vi "Save_Ensight.vi"() -> (5 "Plug in titles":string[](array[string]), 7 "Plug in values":string[](array[string]))   [LabVIEW 2011]
uses:
  Globals/LDA_meas_global_1.vi
  Globals/Plug_in_data_global.vi
  Globals/Meas_global.vi
  Globals/Constants_global.vi
  <vilib>/Analysis/NI_AALBase.lvlib
  <vilib>/ptbypt/NI_PtbyPt.lvlib
panel:
  out "Latest Data":dbl[][](array[numeric])
  out "Variables":dbl[][](array[numeric])
  out "Results File Path":path
  out "Processing first block?":bool
  out "XYZ Position":string[](array[string])
  out "Results File Exists?":bool
  # "You must have just these two indicators on the connector pane of the vi"
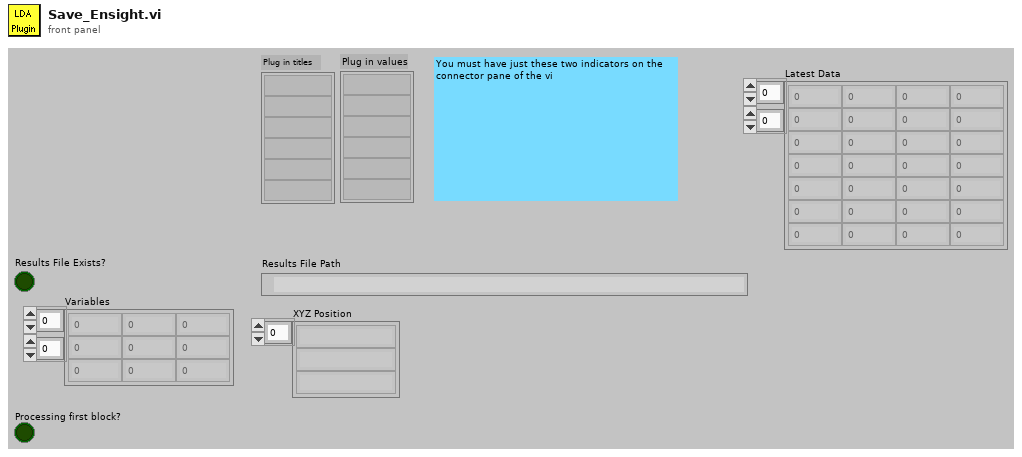
[diagram p1: front panel]
types:
  T1 = typedef "Analysis_info_cluster.ctl" = cluster{"Colour":u32, "Inst type":T2, "Inst name":string, "Symbol":string, "Code name":string, "Extra Info":string, "Inst Array":T3, "Index":i32, "Voltage Index":i32, "Extra Titles":string[], "Extra Values":string[], "Eng Values":dbl[], "Time (ms)":dbl[], "TT / Voltage":dbl[], "u^2":dbl, "U":dbl, "u^3/(u^2)^(1.5)":dbl, "u^4":dbl, "u^4/(u^2)^2 -3":dbl, "Mean % Err":dbl, "% u'/U":dbl}
  T2 = typedef "Inst_type.ctl" = enum16{"Propeller anemometer", "Raw voltage", "Pressure Transducer", "Pitot-static tube", "Preston tube", "Hot wire", "Cross wire 1", "Cross wire 2", "Generic Linear", "Generic Polynomial", "Generic BackPoly", "Fast FID", "Thermocouple", "Cold wire", "Pulsed Wire", "LDA Vel", "LDA Tran time", "LDA Arr time"}
  T3 = typedef "Instrument_Array.ctl" = enum16{"PWA", "LDA", "Analogue"}
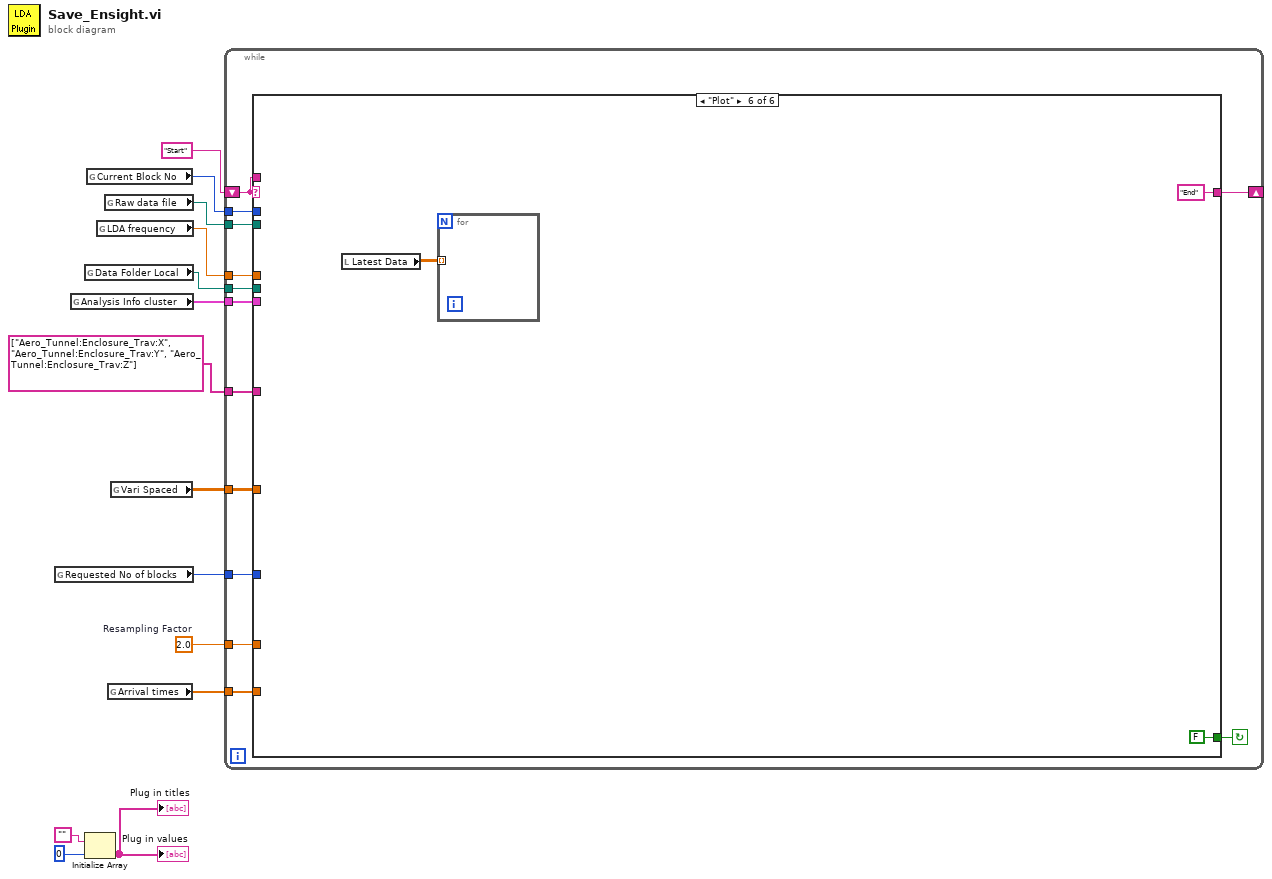
[diagram p0: block diagram]
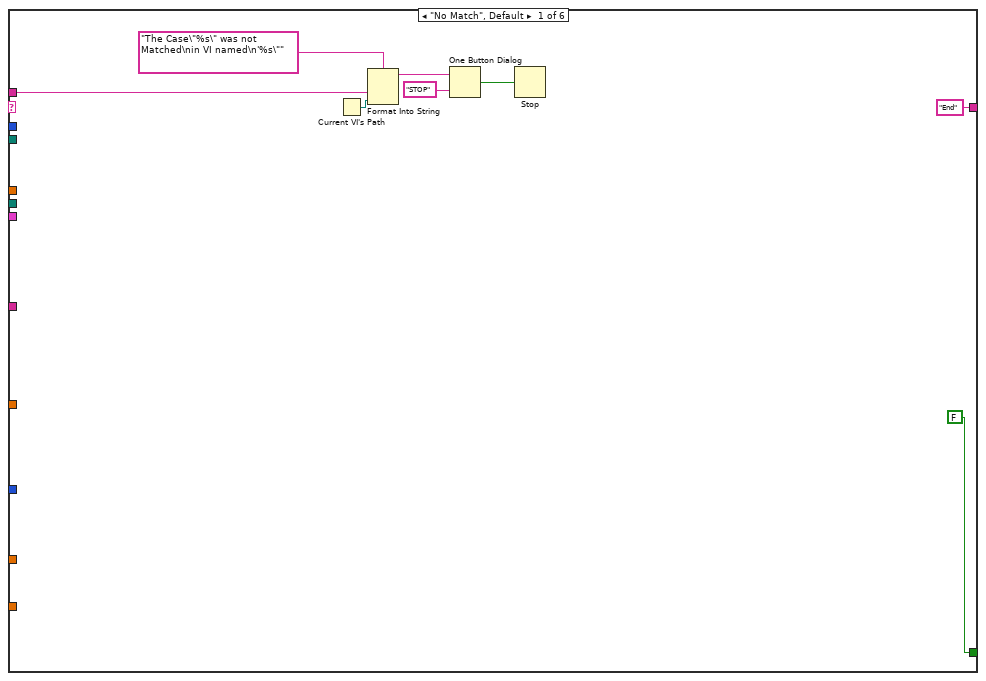
[diagram p2: hidden frame]
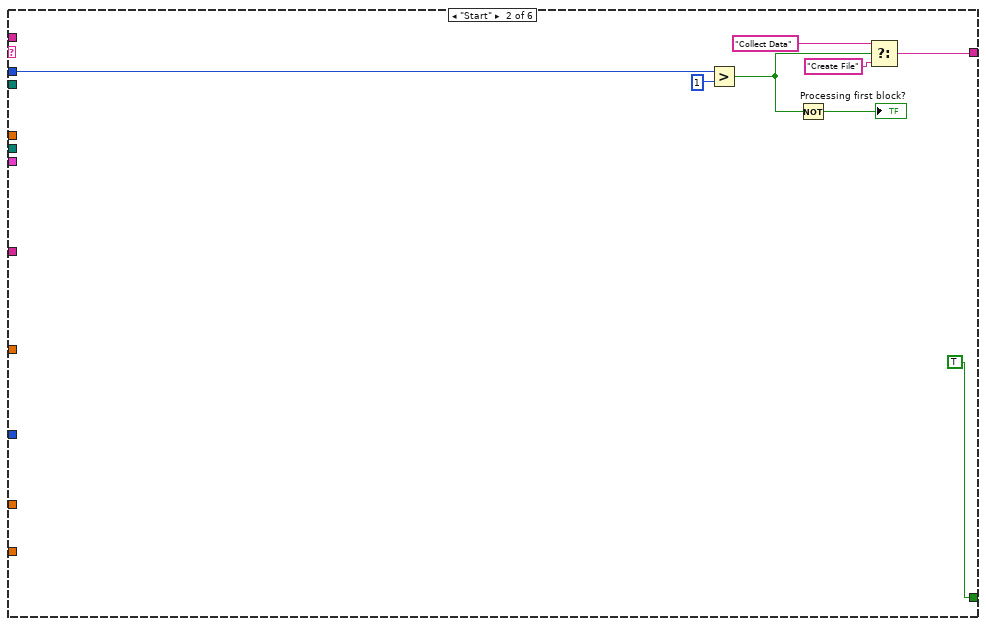
[diagram p3: hidden frame]
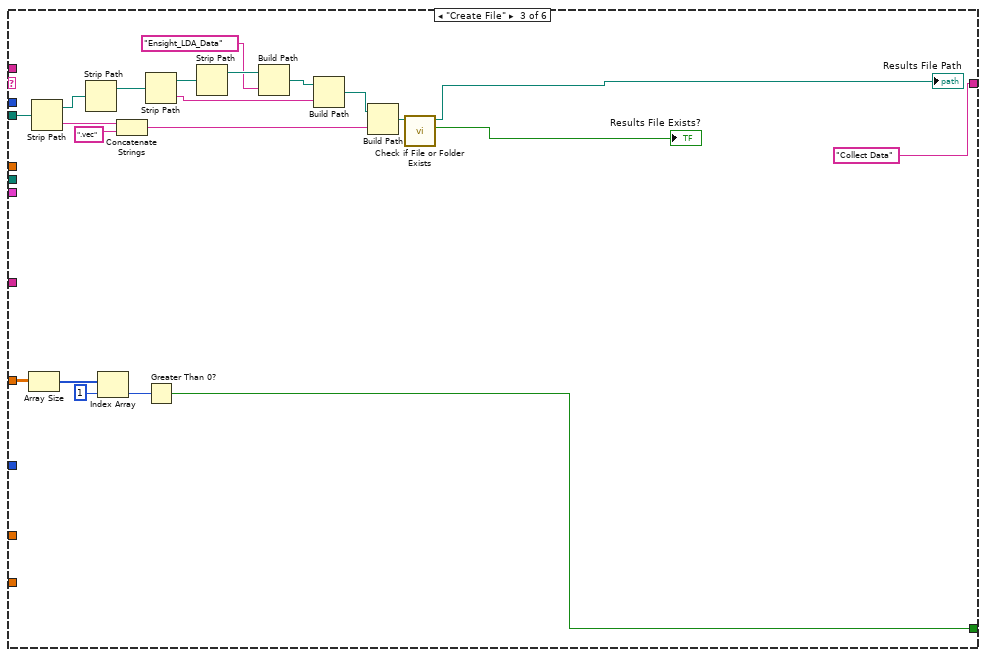
[diagram p4: hidden frame]
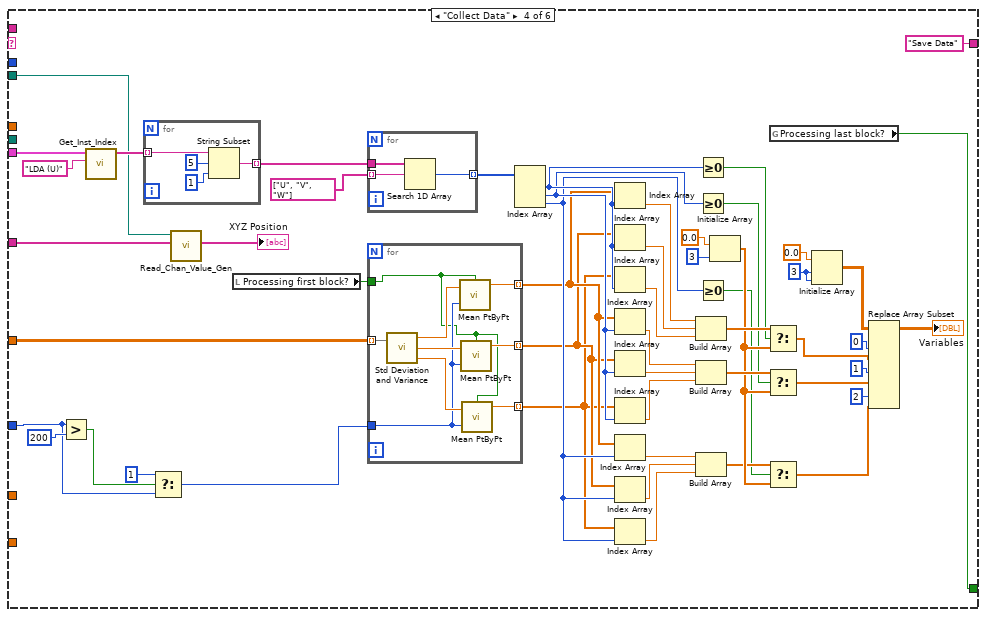
[diagram p5: hidden frame]
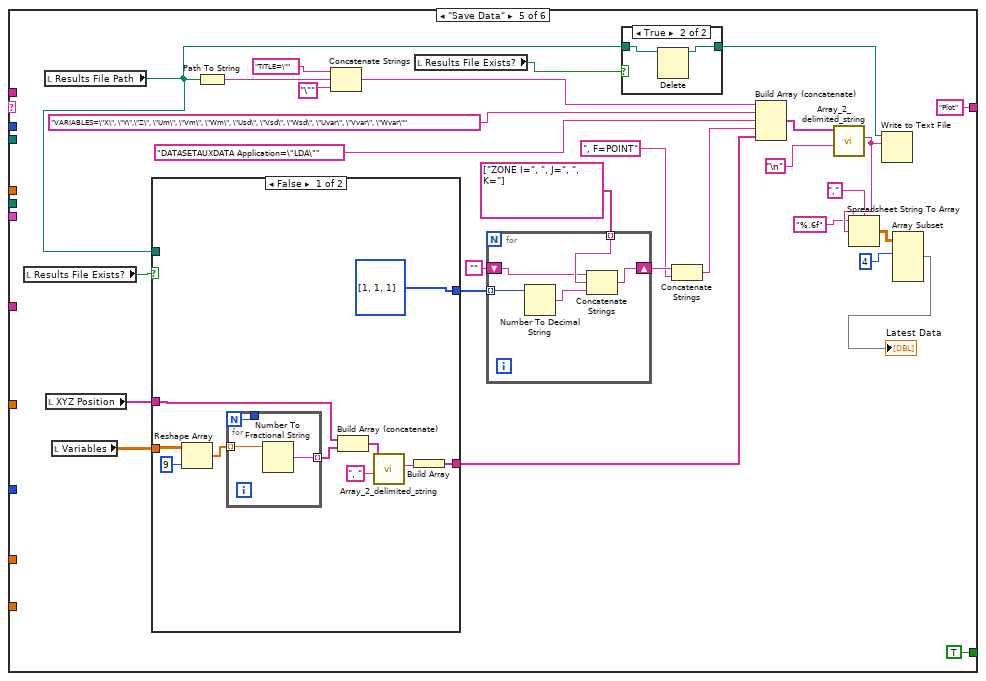
[diagram p6: hidden frame]
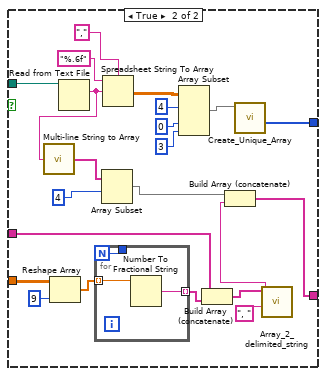
[diagram p8: hidden frame]
diagram:
  w5 = 2.0  # Resampling Factor
  n1 = global read "Meas_global.vi" "Requested No of blocks"() -> (w2:i32)
  n2 = global read "Meas_global.vi" "Analysis Info cluster"() -> (w3:T1[])
  n3 = global read "Constants_global.vi" "Data Folder Local"() -> (w4:path)
  n4 = Initialize Array("", 0) -> (→"Plug in values" →"Plug in titles":string[])
  n5 = global read "Meas_global.vi" "Current Block No"() -> (w8:i32)
  n6 = global read "Meas_global.vi" "LDA frequency"() -> (w6:dbl)
  n7 = global read "Meas_global.vi" "Raw data file"() -> (w7:path)
  n8 = global read "LDA_meas_global_1.vi" "Arrival times"() -> (w12:dbl[])
  n9 = global read "Plug_in_data_global.vi" "Vari Spaced"() -> (w13:dbl[][])
  n10 = while {
    shift-left: "Start" -> [w27]
    shift-right: [w24] -> _
    tunnel: w13 -> [w26]
    tunnel: w12 -> [w25]
    tunnel: w8 -> [w22]
    tunnel: w4 -> [w21]
    tunnel: w7 -> [w20]
    tunnel: w6 -> [w19]
    tunnel: w5 -> [w18]
    tunnel: w3 -> [w17]
    tunnel: w2 -> [w16]
    tunnel: string[] ["Aero_Tunnel:Enclosure_Trav:X", "Aero_Tunnel:Enclosure_Trav:Y", "Aero_Tunnel:Enclosure_Trav:Z"] -> [w15]
    stop <- w23 continue-if-true
    n11 = case shown="\"Plot\"" w27 {
      tunnel: ["End" ("t") w38 "Collect Data" ("t") "Save Data" ("t") "Plot" ("t") "End" ("t")] -> w24
      tunnel: w27 -> [w31 _ _ _ _ _]
      tunnel: w26 -> [_ _ w63 w112 _ _]
      tunnel: w25 -> [_ _ _ _ _ _]
      tunnel: [FALSE TRUE w59 w115 TRUE ("Processing last block?") FALSE ("Processing last block?")] -> w23
      tunnel: w22 -> [_ w37 _ _ _ _]
      tunnel: w21 -> [_ _ _ _ _ _]
      tunnel: w20 -> [_ _ w58 w66 _ _]
      tunnel: w19 -> [_ _ _ _ _ _]
      tunnel: w18 -> [_ _ _ _ _ _]
      tunnel: w17 -> [_ _ _ w113 _ _]
      tunnel: w16 -> [_ _ _ w72 _ _]
      tunnel: w15 -> [_ _ _ w65 _ _]
      frame "No Match", Default {
        n12 = Current VI's Path() -> (path=w30:path)
        n13 = Format Into String(format string="The Case\"%s\" was not Matched\nin VI named\n'%s\"" ("Format String"), w31, w30) -> (resulting string=w34:string)  [unwired: 2 in, 1 out]
        n14 = One Button Dialog(message=w34, button name ("OK")="STOP") -> (true=w32:bool)
        n15 = Stop(stop? (T)=w32) -> ()
      }
      frame "Start" {
        n16 = Greater?(x=w37, y=1) -> (0:w40:bool)
        n17 = Not(x=w40) -> (.not. x?=→"Processing first block?":bool)
        n18 = Select(t="Collect Data", s=w40, f="Create File") -> (s? t:f=w38:string)
      }
      frame "Create File" {
        n19 = Array Size(array=w63) -> (size(s)=w62:i32[])
        n20 = Strip Path(path=w58) -> (stripped path=w57:path, name=w49:string)
        n21 = Strip Path(path=w57) -> (stripped path=w56:path)  [unwired: 1 out]
        n22 = Index Array(array=w62, index=1) -> (element=w60:i32)
        n23 = Concatenate Strings(w49, ".vec" ("string")) -> (w47:string)
        n24 = Strip Path(path=w56) -> (stripped path=w55:path, name=w51:string)
        n25 = Greater Than 0?(x=w60) -> (x > 0?=w59:bool)
        n26 = Strip Path(path=w55) -> (stripped path=w54:path)  [unwired: 1 out]
        n27 = Build Path(base path=w54, name or relative path="Ensight_LDA_Data") -> (appended path=w52:path)
        n28 = Build Path(base path=w52, name or relative path=w51) -> (appended path=w50:path)
        n29 = Build Path(base path=w50, name or relative path=w47) -> (appended path=w46:path)
        n30 = call <vilib>:"Check if File or Folder Exists.vi"("path"=w46) -> ("file or folder exists?"=→"Results File Exists?":bool, "dup path"=→"Results File Path":path)  [unwired: 8 in, 1 out]
      }
      frame "Collect Data" {
        w106 = 3 ("dimension size")
        n31 = Greater?(x=w72, y=200) -> (0:w74:bool)
        n32 = call "Get_Inst_Index.vi"("Inst name search"="LDA (U)", "Analysis Info cluster"=w113) -> ("Inst Name Array"=w110:string[])  [unwired: 7 in, 2 out]
        n33 = for {
          tunnel: w110 -> [w123] mode=indexing
          tunnel: [w120] -> w109 mode=indexing
          n34 = String Subset(string=w123, offset (0)=5, length (rest)=1 ("length (rest)")) -> (substring=w120:string)
        }
        n35 = Select(t=1, s=w74, f=w72) -> (s? t:f=w71:i32)
        n36 = call "Read_Chan_Value_Gen.vi"("Desired Ch Names"=w65, "Raw data file"=w66) -> ("Values"=→"XYZ Position":string[])  [unwired: 9 in]
        n37 = local read "Processing first block?"() -> (w111:bool)
        n38 = for {
          tunnel: w109 -> [w119]
          tunnel: string[] ["U", "V", "W"] -> [w118] mode=indexing
          tunnel: [w117] -> w104 mode=indexing
          n39 = Search 1D Array(1D array=w119, element=w118) -> (index of element=w117:i32)  [unwired: 1 in]
        }
        n40 = for {
          tunnel: w112 -> [w132] mode=indexing
          tunnel: [w128] -> w80 mode=indexing
          tunnel: [w127] -> w79 mode=indexing
          tunnel: [w126] -> w78 mode=indexing
          tunnel: w111 -> [w124]
          tunnel: w71 -> [w125]
          n41 = call <vilib>:"Std Deviation and Variance.vi"("X"=w132) -> ("mean"=w131:dbl, "standard deviation"=w130:dbl, "variance"=w129:dbl)  [unwired: 1 in]
          n42 = call <vilib>:"Mean PtByPt.vi"("x"=w131, "sample length"=w125, "initialize"=w124) -> ("mean"=w128:dbl)  [unwired: 1 in, 1 out]
          n43 = call <vilib>:"Mean PtByPt.vi"("x"=w130, "sample length"=w125, "initialize"=w124) -> ("mean"=w127:dbl)  [unwired: 1 in, 1 out]
          n44 = call <vilib>:"Mean PtByPt.vi"("x"=w129, "sample length"=w125, "initialize"=w124) -> ("mean"=w126:dbl)  [unwired: 1 in, 1 out]
        }
        n45 = Index Array(array=w104) -> (element #1=w102:i32, element #2=w97:i32, element #3=w81:i32)  [unwired: 3 in]
        n46 = Index Array(array=w80, index=w102) -> (element=w101:dbl)
        n47 = Index Array(array=w79, index=w102) -> (element=w100:dbl)
        n48 = Index Array(array=w78, index=w102) -> (element=w99:dbl)
        n49 = Index Array(array=w80, index=w97) -> (element=w94:dbl)
        n50 = Index Array(array=w79, index=w97) -> (element=w93:dbl)
        n51 = Index Array(array=w78, index=w97) -> (element=w92:dbl)
        n52 = Index Array(array=w80, index=w81) -> (element=w82:dbl)
        n53 = Index Array(array=w79, index=w81) -> (element=w83:dbl)
        n54 = Index Array(array=w78, index=w81) -> (element=w84:dbl)
        n55 = Build Array(w101, w100, w99) -> (w98:dbl[])
        n56 = Build Array(w94, w93, w92) -> (w91:dbl[])
        n57 = Build Array(w82, w83, w84) -> (w77:dbl[])
        n58 = Greater Or Equal To 0?(x=w102) -> (x >= 0?=w68:bool)
        n59 = Greater Or Equal To 0?(x=w97) -> (x >= 0?=w69:bool)
        n60 = Greater Or Equal To 0?(x=w81) -> (x >= 0?=w70:bool)
        n61 = Initialize Array(0.0 ("element"), 3 ("dimension size")) -> (w85:dbl[])
        n62 = Select(t=w98, s=w68, f=w85) -> (s? t:f=w90:dbl[])
        n63 = Select(t=w91, s=w69, f=w85) -> (s? t:f=w87:dbl[])
        n64 = Select(t=w77, s=w70, f=w85) -> (s? t:f=w86:dbl[])
        n65 = global read "Meas_global.vi" "Processing last block?"() -> (w115:bool)
        n66 = Initialize Array(0.0 ("element"), w106, w106) -> (w105:dbl[][])
        n67 = Replace Array Subset(array=w105, new element #1=w90, index (col) #1=0 ("disabled index (col)"), new element #2=w87, index (col) #2=1 ("index (col)"), new element #3=w86, index (col) #3=2 ("index (col)")) -> (→"Variables":dbl[][])  [unwired: 3 in]
      }
      frame "Save Data" {
        n68 = local read "Results File Exists?"() -> (w153:bool)
        n69 = local read "Results File Path"() -> (w140:path)
        n70 = local read "XYZ Position"() -> (w134:string[])
        n71 = local read "Variables"() -> (w146:dbl[][])
        n72 = case shown="False" w153 {
          tunnel: w140 -> [_ w197]
          tunnel: [i32[] [1, 1, 1] ("IJK indicies") w196] -> w152
          tunnel: w146 -> [w178 w189]
          tunnel: [w173 w186] -> w145
          tunnel: w134 -> [w171 w184]
          frame False {
            n73 = Reshape Array(w178, 9 ("dimension size")) -> (w176:dbl[])
            n74 = for {
              N -> [w180]
              tunnel: w176 -> [w182] mode=indexing
              tunnel: [w181] -> w172 mode=indexing
              tunnel: [w180] -> _
              n75 = Number To Fractional String(number=w182) -> (F-format string=w181:string)  [unwired: 3 in]
            }
            n76 = Build Array (concatenate)(w171, w172) -> (w170:string[])
            n77 = call "Array_2_delimited_string.vi"("delimiter (Tab)"=", ", "Array of Strings"=w170) -> ("delimited string"=w174:string)  [unwired: 9 in]
            n78 = Build Array(w174) -> (w173:string[])
          }
          frame True {
            n79 = Reshape Array(w189, 9 ("dimension size")) -> (w191:dbl[])
            n80 = Read from Text File(file (use dialog)=w197) -> (text=w195:string)  [unwired: 3 in, 3 out]
            n81 = call "Multi-line String to Array.vi"("Multi lined string"=w195) -> ("Array of string lines"=w194:string[])
            n82 = for {
              N -> [w205]
              tunnel: w191 -> [w207] mode=indexing
              tunnel: [w206] -> w185 mode=indexing
              tunnel: [w205] -> _
              n83 = Number To Fractional String(number=w207) -> (F-format string=w206:string)  [unwired: 3 in]
            }
            n84 = Array Subset(array=w194, index=4) -> (w188:string[])  [unwired: 1 in]
            n85 = Spreadsheet String To Array(delimiter (Tab)=",", format string="%.6f", spreadsheet string=w195) -> (array=w199:dbl[][])  [unwired: 1 in]
            n86 = Array Subset(array=w199, index (row)=4 ("index"), index (col)=0 ("index"), length (col)=3 ("length")) -> (w198:dbl[][])  [unwired: 1 in]
            n87 = Build Array (concatenate)(w184, w185) -> (w183:string[])
            n88 = call "Create_Unique_Array.vi"("2D Array"=w198) -> ("IJK indicies"=w196:i32[])  [unwired: 9 in, 1 out]
            n89 = call "Array_2_delimited_string.vi"("delimiter (Tab)"=", ", "Array of Strings"=w183) -> ("delimited string"=w187:string)  [unwired: 9 in]
            n90 = Build Array (concatenate)(w188, w187) -> (w186:string[])
          }
        }
        n91 = Path To String(path=w140) -> (string=w158:string)
        n92 = Concatenate Strings("TITLE=\"" ("string"), w158, "\"" ("string")) -> (w156:string)
        n93 = local read "Results File Exists?"() -> (w142:bool)
        n94 = for {
          tunnel: w152 -> [w169] mode=indexing
          shift-right: [w167] -> w149
          shift-left: "" -> [w165]
          tunnel: string[] ["ZONE I=", ", J=", ", K="] -> [w166] mode=indexing
          n95 = Number To Decimal String(number=w169) -> (decimal integer string=w168:string)  [unwired: 1 in]
          n96 = Concatenate Strings(w165, w166, w168) -> (w167:string)
        }
        n97 = case shown="True" w142 {
          tunnel: [w162 w163] -> w141
          tunnel: w140 -> [w162 w164]
          frame False {
          }
          frame True {
            n98 = Delete(path (use dialog)=w164) -> (deleted path=w163:path)  [unwired: 4 in, 2 out]
          }
        }
        n99 = Concatenate Strings(w149, ", F=POINT") -> (w147:string)
        n100 = Build Array (concatenate)(w156, "VARIABLES=\"X\", \"Y\",\"Z\", \"Um\", \"Vm\", \"Wm\", \"Usd\", \"Vsd\", \"Wsd\", \"Uvar\", \"Vvar\", \"Wvar\"" ("string"), "DATASETAUXDATA Application=\"LDA\"", w147, w145) -> (w144:string[])
        n101 = call "Array_2_delimited_string.vi"("delimiter (Tab)"="\n", "Array of Strings"=w144) -> ("delimited string"=w137:string)  [unwired: 9 in]
        n102 = Spreadsheet String To Array(delimiter (Tab)=",", format string="%.6f", spreadsheet string=w137) -> (array=w139:dbl[][])  [unwired: 1 in]
        n103 = Write to Text File(file (use dialog)=w141, text=w137) -> ()  [unwired: 2 in, 3 out]
        n104 = Array Subset(array=w139, index (row)=4 ("index")) -> (→"Latest Data":dbl[][])  [unwired: 3 in]
      }
      frame "Plot" {
        n105 = local read "Latest Data"() -> (w208:dbl[][])
        n106 = for {
          tunnel: w208 -> [_] mode=indexing
        }
      }
    }
  }
